vi "IMAQdx Configure Grab.vi"(8 "error in":errorcluster, 11 "Session In":T1) -> (0 "error out":errorcluster, 3 "Session Out":T1)   [LabVIEW 2013, in "NI_Vision_Acquisition_Software.lvlib"]
doc: "Configures and starts a grab acquisition. A grab performs an acquisition that loops continually on a ring of buffers. Use the grab VI for high-speed image acquisition. Use IMAQdx Grab.vi to copy an image out of the buffer. If you call this VI before calling IMAQdx Open Camera.vi, IMAQdx Configure Grab.vi uses cam0 by default. Use IMAQdx Unconfigure Acquisition.vi to unconfigure the acquisition."
uses:
  NI_Vision_Acquisition_Software.lvlib
  IMAQdx.ctl
  IMAQdx Acquisition Mode.ctl
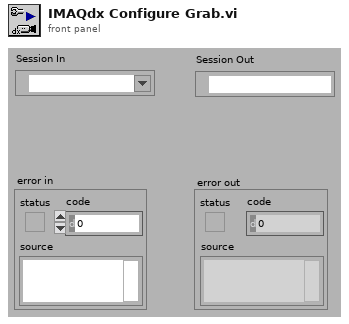
[diagram p1: front panel]
types:
  T1 = typedef "IMAQdx.ctl" = refnum<k21>
  T2 = typedef "NI_Vision_Acquisition_Software.lvlib/IMAQdx Acquisition Mode.ctl" = enum32{"One Shot", "Continuous"}
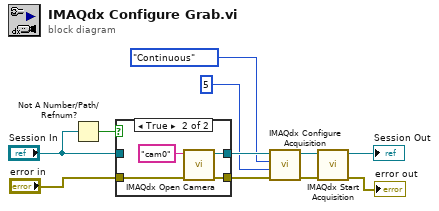
[diagram p0: block diagram]
diagram:
  n1 = Not A Number/Path/Refnum?(number/path/refnum="Session In") -> (NaN/Path/Refnum?=w3:bool)
  n2 = case shown="True" w3 {
    tunnel: [w13 w17] -> w11
    tunnel: "Session In" -> [w13 _]
    tunnel: [w12 w16] -> w9
    tunnel: "error in" -> [w12 w15]
    frame False {
    }
    frame True {
      n3 = call "IMAQdx Open Camera.vi"("error in"=w15, "Session In"="cam0") -> ("error out"=w16:errorcluster, "Session Out"=w17:T1)  [unwired: 8 in]
    }
  }
  n4 = call "IMAQdx Configure Acquisition.vi"("error in"=w9, "Number of Buffers"=u32 5, "Continuous?"=IMAQdx_Acquisition_Mode."Continuous", "Session In"=w11) -> ("error out"=w4:errorcluster, "Session Out"=w5:T1)  [unwired: 6 in]
  n5 = call "IMAQdx Start Acquisition.vi"("error in"=w4, "Session In"=w5) -> ("error out"=→"error out":errorcluster, "Session Out"=→"Session Out":T1)  [unwired: 8 in]
